vi "funcionttt.vi"(0 "Num":dbl[](array[numeric]), 1 "Den":dbl[](array[numeric]), 2 "Retardo":dbl, 3 "XINIT":dbl[](array[numeric]), 4 "DT":dbl, 5 "U":dbl) -> (14 "Y":dbl format="%.2f", 15 "Out":dbl[](array[numeric]))   [LabVIEW 2019]
uses:
  <vilib>/Analysis/Matrix/Datatypes/RealMatrix.ctl
  <vilib>/Analysis/baseanly.llb/Real Dot Product.vi
  <vilib>/Analysis/NI_AALBase.lvlib
  <vilib>/Analysis/Matrix/NI_Matrix.lvlib
panel:
  out "ai":dbl[](array[numeric])
  out "A":T1
  out "Dx":dbl[](array[numeric])
  out "B":dbl[](array[numeric])
  out "n":i32
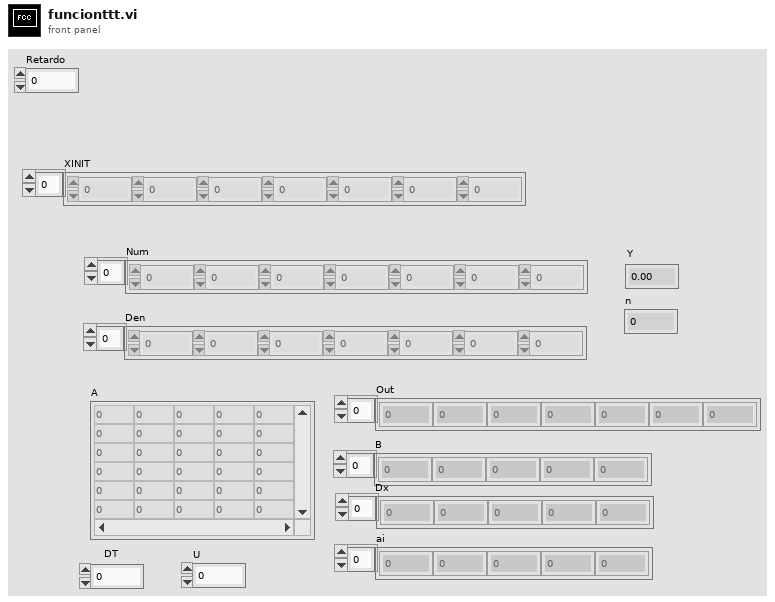
[diagram p1: front panel]
types:
  T1 = typedef "NI_Matrix.lvlib/RealMatrix.ctl" = dbl[][]
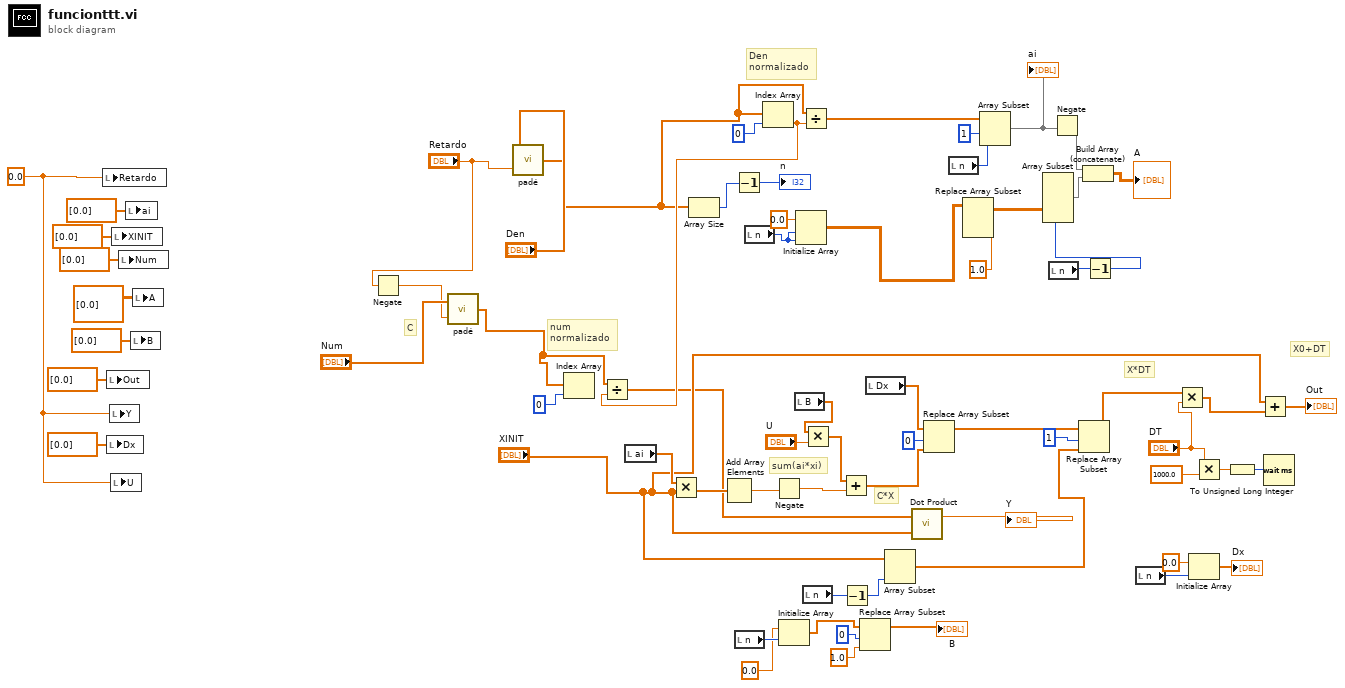
[diagram p0: block diagram]
diagram:
  w8 = 0.0 ("Retardo")
  # "num\nnormalizado"
  # "X0+DT"
  # "C*X"
  # "sum(ai*xi)"
  # "X*DT"
  # "Den\nnormalizado"
  # "C"
  n1 = local write "Retardo"(w8) -> ()
  n2 = local write "Out"(dbl[] [0.0] ("Out")) -> ()
  n3 = local write "Dx"(dbl[] [0.0] ("Dx")) -> ()
  n4 = local write "Y"(w8) -> ()
  n5 = local write "U"(w8) -> ()
  n6 = local write "XINIT"(dbl[] [0.0] ("XINIT")) -> ()
  n7 = local write "Num"(dbl[] [0.0] ("Num")) -> ()
  n8 = local write "ai"(dbl[] [0.0] ("ai")) -> ()
  n9 = local write "B"(dbl[] [0.0] ("B")) -> ()
  n10 = local write "A"(T1 [[0.0]] ("A")) -> ()
  n11 = Negate(x="Retardo") -> (-x=w10:dbl)
  n12 = call "padé.vi"("Retardo"=w10, "Num\n Den"="Num") -> ("Salida"=w9:dbl[])
  n13 = call "padé.vi"("Retardo"="Retardo", "Num\n Den"="Den") -> ("Salida"=w13:dbl[])
  n14 = Index Array(array=w9, index=0) -> ()  [unwired: 1 out]
  n15 = local read "ai"() -> (w50:dbl[])
  n16 = Multiply(x=w50, y="XINIT") -> (x*y=w49:dbl[])
  n17 = Array Size(array=w13) -> (size(s)=w65:i32)
  n18 = Add Array Elements(numeric array=w49) -> (sum=w48:dbl)
  n19 = Decrement(x=w65) -> (x-1=→"n":i32)
  n20 = local read "n"() -> (w24:i32)
  n21 = local read "n"() -> (w64:i32)
  n22 = Index Array(array=w13, index=0) -> (element=w16:dbl)
  n23 = Divide(x=w9, y=w16) -> (x/y=w15:dbl[])
  n24 = Negate(x=w48) -> (-x=w47:dbl)
  n25 = Initialize Array(0.0 ("element"), w24) -> (w25:dbl[])
  n26 = local read "B"() -> (w45:dbl[])
  n27 = Initialize Array(0.0 ("element"), w64, w64) -> (w67:dbl[][])
  n28 = Divide(x=w13, y=w16) -> (x/y=w51:dbl[])
  n29 = Multiply(x=w45, y="U") -> (x*y=w44:dbl[])
  n30 = local read "n"() -> (w43:i32)
  n31 = Add(x=w44, y=w47) -> (x+y=w39:dbl[])
  n32 = Decrement(x=w43) -> (x-1=w42:i32)
  n33 = Replace Array Subset(array=w25, new element=1.0 ("new element/subarray"), index=0) -> (→"B":dbl[])
  n34 = local read "Dx"() -> (w38:dbl[])
  n35 = Array Subset(array="XINIT", length=w42) -> (w35:dbl[])  [unwired: 1 in]
  n36 = call-poly <vilib>:"Dot Product.vi"("Y Vector"="XINIT", "X Vector"=w15) -> ("X * Y"=→"Y":dbl)  [unwired: 1 out]
  n37 = Replace Array Subset(array=w38, new element=w39, index=0) -> (w37:dbl[])
  n38 = local read "n"() -> (w59:i32)
  n39 = Replace Array Subset(array=w67, new element=1.0 ("new diagonal/fill element")) -> (w61:T1)  [unwired: 2 in]
  n40 = Array Subset(array=w51, index=1, length=w59) -> (w57:dbl[])
  "ai" <- w57
  n41 = local read "n"() -> (w60:i32)
  n42 = Negate(x=w57) -> (-x=w55:dbl[])
  n43 = Replace Array Subset(array=w37, new element=w35, index=1) -> (w31:dbl[])
  n44 = Decrement(x=w60) -> (x-1=w56:i32)
  n45 = Array Subset(array=w61, length (row)=w56) -> (w54:T1)  [unwired: 3 in]
  n46 = Build Array (concatenate)(w55, w54) -> (→"A":T1)
  n47 = local read "n"() -> (w26:i32)
  n48 = Multiply(x=w31, y="DT") -> (x*y=w29:dbl[])
  n49 = Initialize Array(0.0 ("element"), w26) -> (→"Dx":dbl[])
  n50 = Multiply(x="DT", y=1000.0) -> (x*y=w33:dbl)
  n51 = To Unsigned Long Integer(number=w33) -> (unsigned 32bit integer=w32:u32)
  n52 = Add(x="XINIT", y=w29) -> (x+y=→"Out":dbl[])
  n53 = Wait (ms)(milliseconds to wait=w32) -> ()  [unwired: 1 out]
